vi "CC Script Check Telescope is Close Enough.vi"(7 "Target Object":string, 10 "Current Pos":T1, 11 "Target Pos":T1) -> (1 "msg":string, 2 "In Range?":cluster{"RA":bool, "DEC":bool}, 3 "close enough":bool)   [LabVIEW 2024]
uses:
  typedefs/CC cluster RA and DEC.ctl
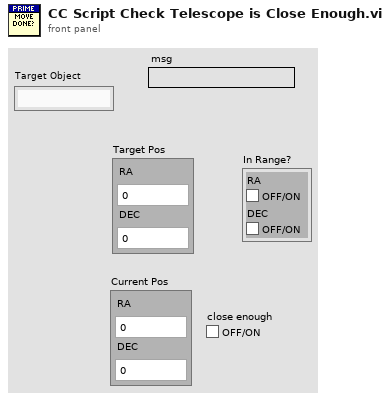
[diagram p1: front panel]
types:
  T1 = typedef "CC cluster RA and DEC.ctl" = cluster{"RA":dbl, "DEC":dbl}
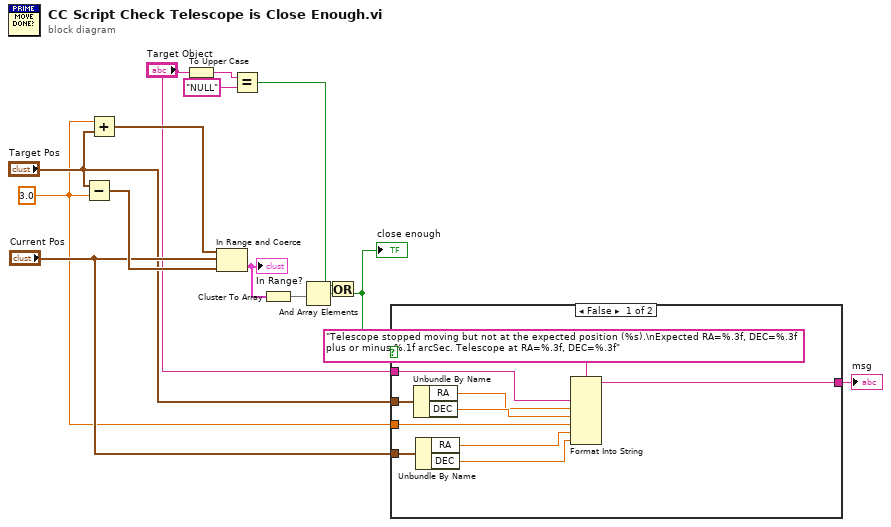
[diagram p0: block diagram]
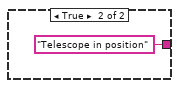
[diagram p2: hidden frame]
diagram:
  w6 = 3.0
  n1 = Subtract(x="Target Pos", y=w6) -> (x-y=w14:T1)
  n2 = Add(x=w6, y="Target Pos") -> (x+y=w11:T1)
  n3 = To Upper Case(1:"Target Object") -> (0:w5:string)
  n4 = In Range and Coerce(upper limit=w11, x="Current Pos", lower limit=w14) -> (In Range?=w13:cluster{"RA":bool, "DEC":bool})  [unwired: 1 out]
  "In Range?" <- w13
  n5 = Equal?(x=w5, y="NULL") -> (x = y?=w2:bool)
  n6 = Cluster To Array(cluster=w13) -> (array=w12:bool[])
  n7 = And Array Elements(Boolean array=w12) -> (logical AND=w9:bool)
  n8 = Or(x=w2, y=w9) -> (x .or. y?=w3:bool)
  "close enough" <- w3
  n9 = case shown="False" w3 {
    tunnel: "Target Pos" -> [w23 _]
    tunnel: "Current Pos" -> [w21 _]
    tunnel: [w18 "Telescope in position"] -> w8
    tunnel: w6 -> [w17 _]
    tunnel: "Target Object" -> [w15 _]
    frame False {
      n10 = Unbundle By Name(w23) -> ("RA"=w16:dbl, "DEC"=w22:dbl)
      n11 = Unbundle By Name(w21) -> ("RA"=w20:dbl, "DEC"=w19:dbl)
      n12 = Format Into String(format string="Telescope stopped moving but not at the expected position (%s).\nExpected RA=%.3f, DEC=%.3f plus or minus %.1f arcSec. Telescope at RA=%.3f, DEC=%.3f" ("Message"), w15, w16, w22, w17, w20, w19) -> (resulting string=w18:string)  [unwired: 2 in, 1 out]
    }
    frame True {
    }
  }
  "msg" <- w8
